vi "Write Startup Launch Nested Views Msg.vi"(10 "Launch Nested Views Msg":refnum<class "Launch Nested Views Msg.lvclass">, 11 "IViewManager in":refnum<class "IViewManager.lvclass">) -> (3 "IViewManager out":refnum<class "IViewManager.lvclass">)   [LabVIEW 2018, in "MVA Framework.lvlib" / "IViewManager.lvlib" / "IViewManager.lvclass"]
doc: "写入启动启动嵌套视图消息"
uses:
  IViewManager.lvclass
  IViewManager Messages/Launch Nested Views Msg/Launch Nested Views Msg.lvclass
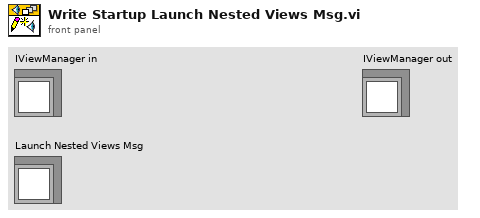
[diagram p1: front panel]
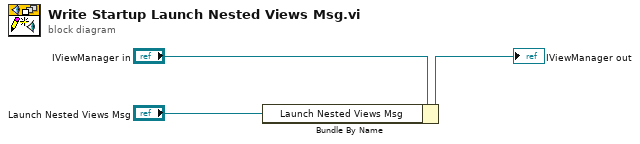
[diagram p0: block diagram]
diagram:
  n1 = Bundle By Name(cluster="IViewManager in", "Launch Nested Views Msg"="Launch Nested Views Msg") -> (→"IViewManager out":refnum<class "IViewManager.lvclass">)
